vi "RT Network Stream Endpoints.vi"() -> ()   [LabVIEW 2014]
uses:
  controls/UI Data.ctl
panel:
  in  "NS Error Writer":refnum<k21>
  out "NS Command Reader":refnum<k21>
  # "The NS Error Writer control was created from the writer endpoint terminal of a Create Network Stream Writer Endpoint function with a data type of UI Data.ctl (typedef)."
  # "The NS Command Reader control was created from the reader endpoint terminal of a Create Network Stream Reader Endpoint function with a data type of UI Data.ctl (typedef)."
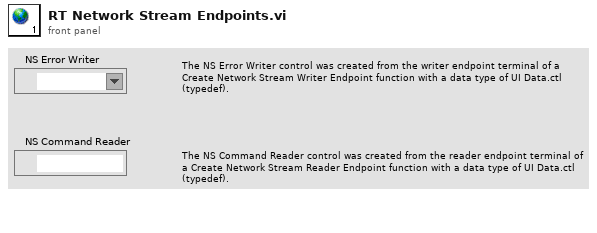
[diagram p1: front panel]
diagram:
